vi "Compare_Calculate_TargetOffsets.vi"() -> ()   [LabVIEW 2019]
panel:
  in  "distance":dbl
  in  "depth":dbl
  out "Numeric":i32
  out "Test Plot":cluster{dbl[], dbl[]}[](graph)
  in  "StopValue":dbl=300.0
  in  "StartValue":dbl
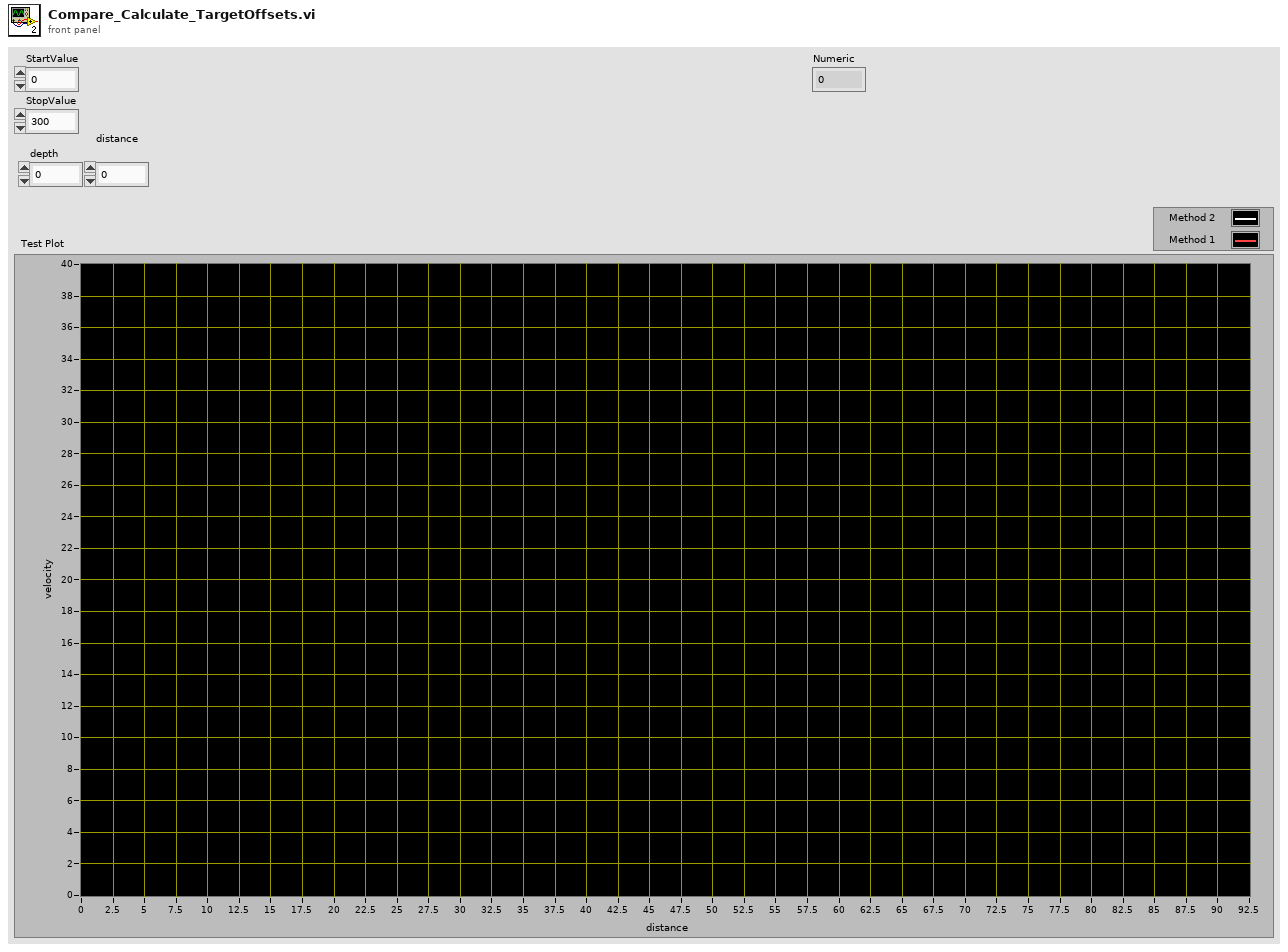
[diagram p1: front panel]
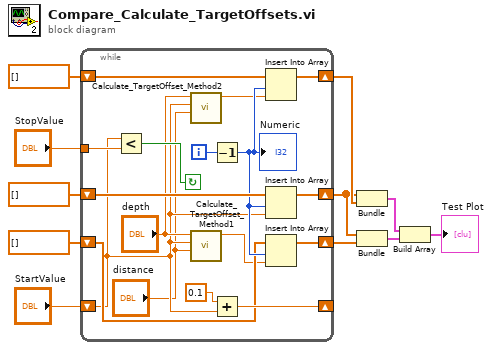
[diagram p0: block diagram]
diagram:
  n1 = while {
    shift-right: [w27] -> _
    shift-left: "StartValue" -> [w15]
    tunnel: "StopValue" -> [w26]
    shift-right: [w21] -> w5
    shift-left: dbl[] [] -> [w23]
    shift-right: [w20] -> w7
    shift-left: dbl[] [] -> [w22]
    shift-right: [w17] -> w4
    shift-left: dbl[] [] -> [w18]
    i -> [w24]
    stop <- w25 continue-if-true
    n2 = Less?(x=w15, y=w26) -> (x < y?=w25:bool)
    n3 = call "Calculate_TargetOffset_Method2.vi"("distance"="distance", "skew"=w15, "depth"="depth") -> ("target offset"=w12:dbl)  [unwired: 7 in, 1 out]
    n4 = call "Calculate_TargetOffset_Method1.vi"("distance"="distance", "skew"=w15, "depth"="depth") -> ("target offset"=w13:dbl)  [unwired: 7 in, 1 out]
    n5 = Decrement(x=w24) -> (x-1=w19:i32)
    "Numeric" <- w19
    n6 = Add(x=0.1, y=w15) -> (x+y=w27:dbl)
    n7 = Insert Into Array(array=w22, index=w19, new element=w12) -> (w20:dbl[])
    n8 = Insert Into Array(array=w23, index=w19, new element=w15) -> (w21:dbl[])
    n9 = Insert Into Array(array=w18, index=w19, new element=w13) -> (w17:dbl[])
  }
  n10 = Bundle(w5, w7) -> (w3:cluster{dbl[], dbl[]})  [unwired: 1 in]
  n11 = Bundle(w5, w4) -> (w2:cluster{dbl[], dbl[]})  [unwired: 1 in]
  n12 = Build Array(w3, w2) -> (→"Test Plot":cluster{dbl[], dbl[]}[])
